vi "SerialClient.vi"(0 "Format":enum32{"RTU", "ASCII"}(ring), 1 "Port":string(combo)="COM3", 2 "Baudrate":i32(ring)=19200 items=["4800"=4800, "9600"=9600, "19200"=19200, "38400"=38400, "57600"=57600, "115200"=115200], 3 "Parity":string(combo)="E", 4 "Data Bits":i32(ring)=8 items=["7"=7, "8"=8], 5 "Stop Bits":i32(ring)=1 items=["1"=1, "2"=2], 7 "Flow":enum32{"NONE", "RTS/CTS"}(ring)) -> (12 "error out":errorcluster, 14 "Handle Out":u64[](array[numeric]))   [LabVIEW 2020, in "SnapMB.lvlib"]
uses:
  SnapMB.lvlib
  windows/snapmb.dll
panel:
  in  "error in (no error)":errorcluster
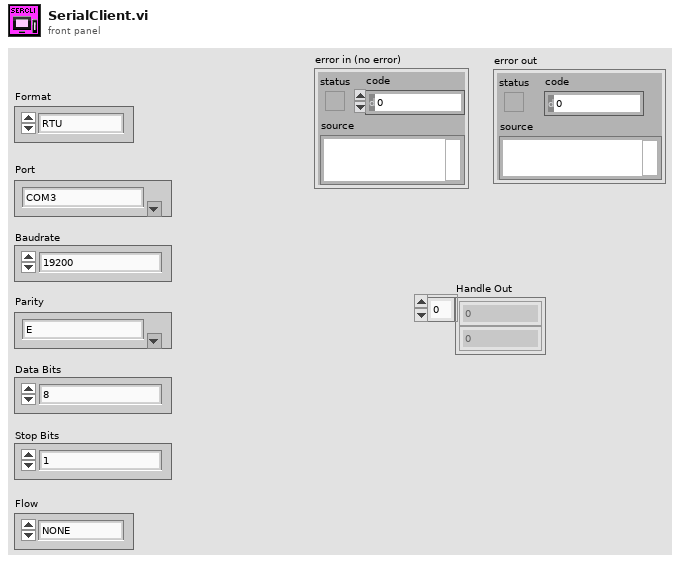
[diagram p1: front panel]
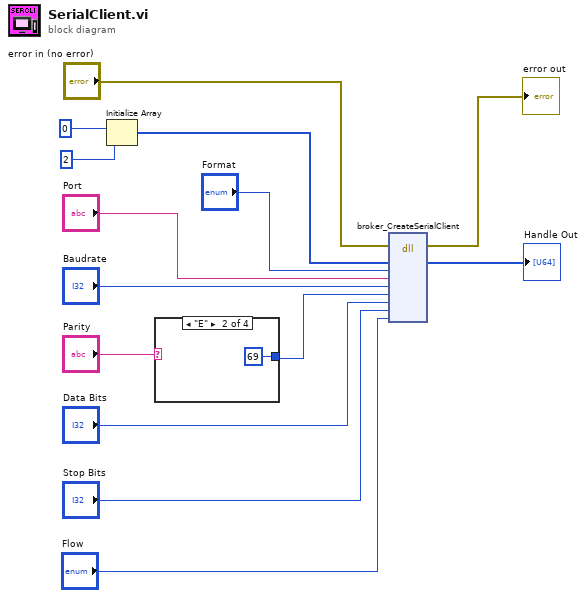
[diagram p0: block diagram]
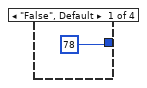
[diagram p2: hidden frame]
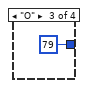
[diagram p3: hidden frame]
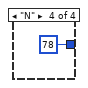
[diagram p4: hidden frame]
diagram:
  n1 = Initialize Array(u64 0 ("element"), 2 ("dimension size")) -> (w5:u64[])
  n2 = case shown="\"E\"" "Parity" {
    tunnel: [u8 78 ("Parity") u8 69 ("Parity") u8 79 ("Parity") u8 78 ("Parity")] -> w1
    frame "False", Default {
    }
    frame "E" {
    }
    frame "O" {
    }
    frame "N" {
    }
  }
  n3 = dll-call lib="D:/SnapMB/LabVIEW/lib/windows/snapmb.dll" fn="broker_CreateSerialClient"(error in="error in (no error)", "Handle"=w5, "Format"="Format", "Port"="Port", "Baudrate"="Baudrate", "Parity"=w1, "Data Bits"="Data Bits", "Stop Bits"="Stop Bits", "Flow"="Flow") -> (error out=→"error out":errorcluster, "Handle"=→"Handle Out":u64[])  [unwired: 10 in, 1 out]
